vi "Parse Mail Box Status.vi"(11 "status":u8) -> (3 "Status Meaning":string)   [LabVIEW 2017, in "NI_Robotics_KUKA youBot Host.lvlib"]
uses:
  <vilib>/robotics/KUKA youBot/NI_Robotics_KUKA youBot Host.lvlib
  <vilib>/robotics/KUKA youBot/KUKA youBot Global Value.vi
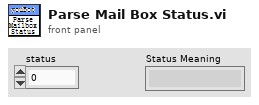
[diagram p1: front panel]
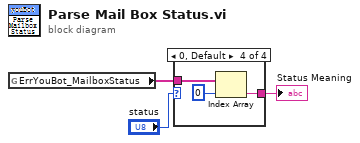
[diagram p0: block diagram]
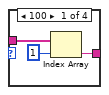
[diagram p2: hidden frame]
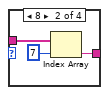
[diagram p3: hidden frame]
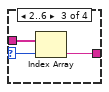
[diagram p4: hidden frame]
diagram:
  n1 = global read "KUKA youBot Global Value.vi" "ErrYouBot_MailboxStatus"() -> (w2:string[])
  n2 = case shown="0, Default" "status" {
    selector: "status" -> [_ _ w11 _]
    tunnel: w2 -> [w6 w9 w12 w15]
    tunnel: [w4 w7 w10 w13] -> w1
    frame 100 {
      n3 = Index Array(array=w6, index=1) -> (element=w4:string)
    }
    frame 8 {
      n4 = Index Array(array=w9, index=7) -> (element=w7:string)
    }
    frame 2..6 {
      n5 = Index Array(array=w12, index=w11) -> (element=w10:string)
    }
    frame 0, Default {
      n6 = Index Array(array=w15, index=0) -> (element=w13:string)
    }
  }
  "Status Meaning" <- w1
